vi "Read Sources.vi"(8 "error in (no error)":errorcluster, 11 "DigitizerBase in":refnum<class "DigitizerBase.lvclass">) -> (0 "error out":errorcluster, 2 "Sources":T1[](array[typedef]), 3 "DigitizerBase out":refnum<class "DigitizerBase.lvclass">)   [LabVIEW 2014, in "DigitizerPlugins.lvlib" / "DigitizerBase.lvclass"]
uses:
  DigitizerBase.lvclass
  Typedefs/TrigSource.ctl
  DigitizerBase.lvclass/DigitizerBase.ctl
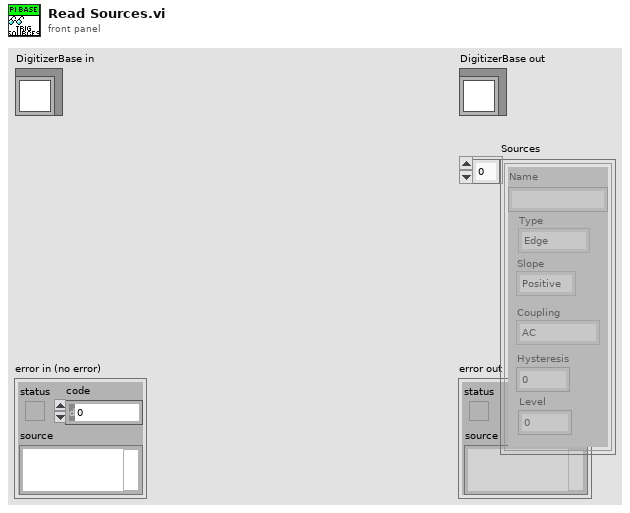
[diagram p1: front panel]
types:
  T1 = typedef "DigitizerPlugins.lvlib/DigitizerBase.lvclass/TrigSource.ctl" = cluster{"Name":string, "Coupling":enum16{"AC", "DC", "HF Reject", "LF Reject", "Noise Reject"}, "Hysteresis":dbl, "Level":dbl, "Slope":enum16{"Positive", "Negative"}, "Type":enum16{"Edge", "Width", "Runt", "Glitch", "TV", "Window"}}
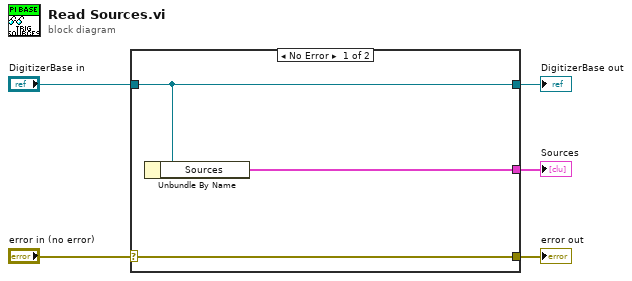
[diagram p0: block diagram]
diagram:
  n1 = case shown="No Error" "error in (no error)" {
    selector: "error in (no error)" -> [w8 w9]
    tunnel: [w8 w9] -> w4
    tunnel: [w7 w10] -> w2
    tunnel: "DigitizerBase in" -> [w7 w10]
    tunnel: [w6 _] -> w1
    frame No Error {
      n2 = Unbundle By Name(w7) -> ("Sources"=w6:T1[])
    }
    frame Error {
    }
  }
  "error out" <- w4
  "DigitizerBase out" <- w2
  "Sources" <- w1
